vi "readLogServoLoops.vi"(8 "error in (no error)":errorcluster, 10 "Parser":refnum<class "U8ArrayParserAutoIndexing.lvclass">, 11 "M1M3SAL in":refnum<class "M1M3SAL.lvclass">) -> (0 "error out":errorcluster, 2 "EventServoLoops":variant, 3 "M1M3SAL out":refnum<class "M1M3SAL.lvclass">)   [LabVIEW 2016, in "M1M3SupportCommunicator.lvlib" / "M1M3SAL.lvclass"]
uses:
  M1M3SAL.lvclass
  Common_RT_Utilities/U8ArrayParserAutoIndexing/U8ArrayParserAutoIndexing.lvclass
  DataTypes/Topics/EventServoLoops.ctl
  DataTypes/Topics/Parts/Timestamp.ctl
  DataTypes/Topics/M1M3SupportTopics.lvlib
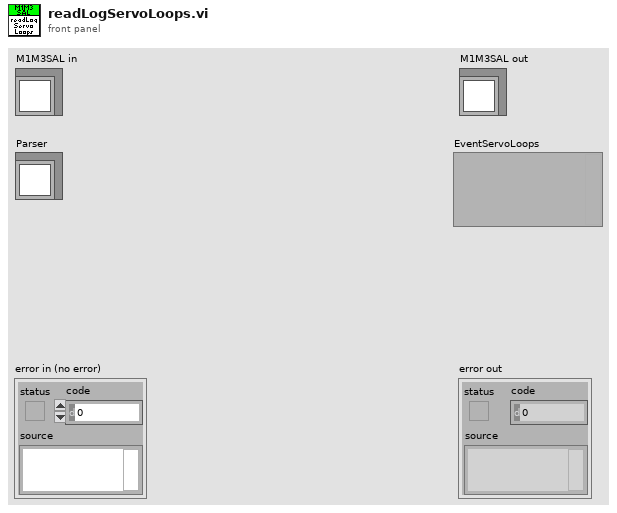
[diagram p1: front panel]
types:
  T1 = typedef "M1M3SupportTopics.lvlib/EventServoLoops.ctl" = cluster{"Timestamp":T2, "HardpointChase":bool, "HardpointOffloading":bool, "OuterLoopTimeOk":bool}
  T2 = typedef "M1M3SupportTopics.lvlib/Timestamp.ctl" = dbl
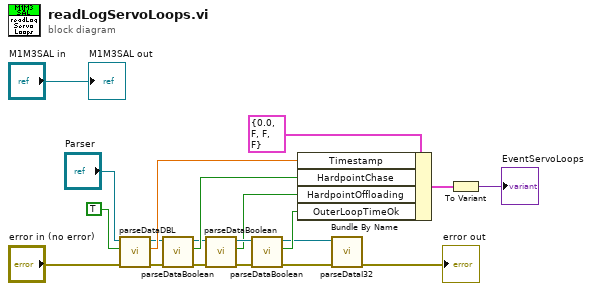
[diagram p0: block diagram]
diagram:
  n1 = call "parseDataDBL.vi"("error in (no error)"="error in (no error)", "OverrideSwapBytes"=TRUE, "U8ArrayParserAutoIndexing in"="Parser") -> ("error out"=w11:errorcluster, "Data"=w13:dbl, "U8ArrayParserAutoIndexing out"=w12:refnum<class "U8ArrayParserAutoIndexing.lvclass">)  [unwired: 6 in]
  n2 = call "parseDataBoolean.vi"("error in (no error)"=w11, "U8ArrayParserAutoIndexing in"=w12) -> ("error out"=w7:errorcluster, "Data"=w10:bool, "U8ArrayParserAutoIndexing out"=w8:refnum<class "U8ArrayParserAutoIndexing.lvclass">)  [unwired: 7 in]
  n3 = call "parseDataBoolean.vi"("error in (no error)"=w7, "U8ArrayParserAutoIndexing in"=w8) -> ("error out"=w6:errorcluster, "Data"=w4:bool, "U8ArrayParserAutoIndexing out"=w5:refnum<class "U8ArrayParserAutoIndexing.lvclass">)  [unwired: 7 in]
  n4 = call "parseDataBoolean.vi"("error in (no error)"=w6, "U8ArrayParserAutoIndexing in"=w5) -> ("error out"=w1:errorcluster, "Data"=w3:bool, "U8ArrayParserAutoIndexing out"=w2:refnum<class "U8ArrayParserAutoIndexing.lvclass">)  [unwired: 7 in]
  n5 = Bundle By Name(cluster=T1 {"Timestamp"=0.0, "HardpointChase"=FALSE, "HardpointOffloading"=FALSE, "OuterLoopTimeOk"=FALSE} ("EventServoLoops"), "Timestamp"=w13, "HardpointChase"=w10, "HardpointOffloading"=w4, "OuterLoopTimeOk"=w3) -> (w19:T1)
  n6 = call "parseDataI32.vi"("error in (no error)"=w1, "U8ArrayParserAutoIndexing in"=w2) -> ("error out"=→"error out":errorcluster)  [unwired: 7 in, 2 out]
  n7 = To Variant(anything=w19) -> (Variant=→"EventServoLoops":variant)
  "M1M3SAL out" <- "M1M3SAL in"
